vi "ZCR_measurement_loader.vi"() -> ()   [LabVIEW 2020, in "Library Commun.lvlib" / "Nodon_ZCR.lvclass"]
uses:
  Nodon_ZCR.lvclass
  <vilib>/Waveform/WDTFileIO.llb/Read Waveform from File.vi
panel:
  out "Waveform Graph":waveform(dbl)[](graph)
  in  "Path":path
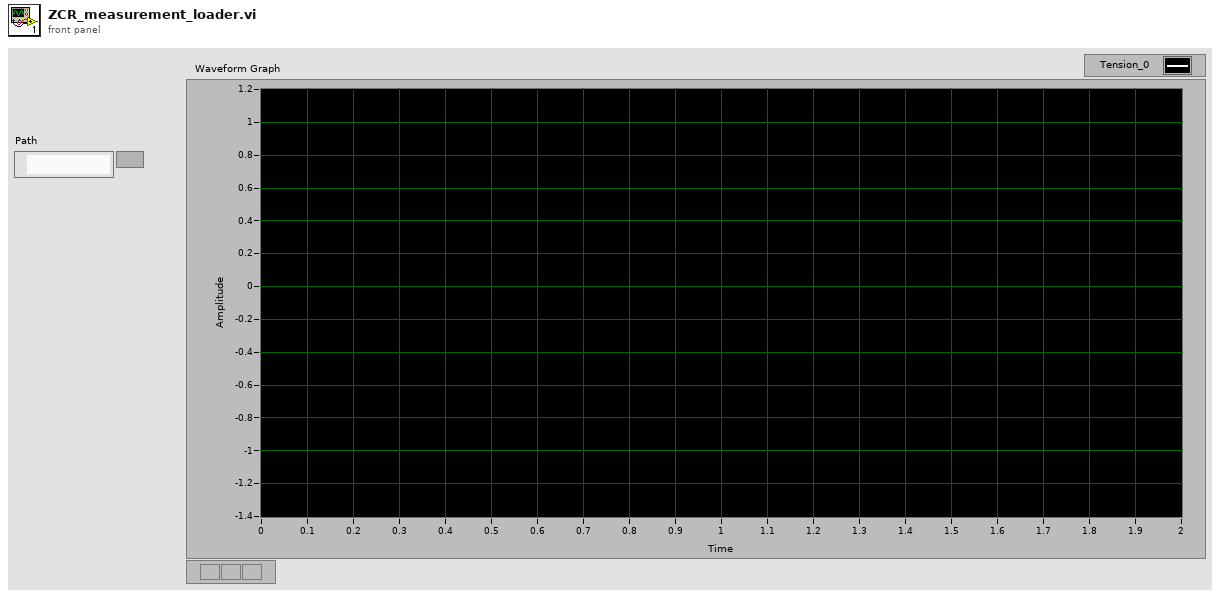
[diagram p1: front panel]
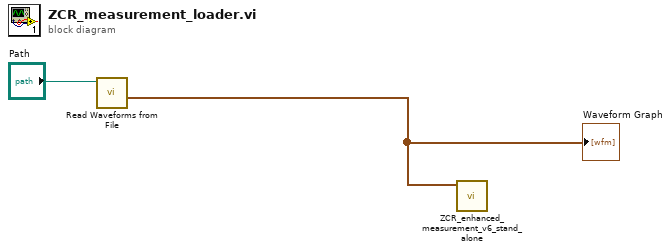
[diagram p0: block diagram]
diagram:
  n1 = call-poly <vilib>:"Read Waveforms from File.vi"("file path (dialog if empty)"="Path") -> ("all waveforms in record"=w1:waveform(dbl)[])  [unwired: 5 in, 3 out]
  "Waveform Graph" <- w1
  n2 = call "ZCR_enhanced_measurement_v6_stand_alone.vi"("ZCR Signal Input"=w1) -> ()  [unwired: 6 in, 5 out]
